vi "ADC Read Current.vi"(4 "Range":string, 8 "Bit depth":u8 max=3 step=1, 11 "VISA Refnum in":refnum<visa-resource-name>) -> (0 "Current in uA":dbl, 1 "Configuration byte":u8, 3 "VISA Refnum out":refnum<visa-resource-name>)   [LabVIEW 2015]
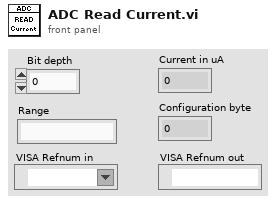
[diagram p1: front panel]
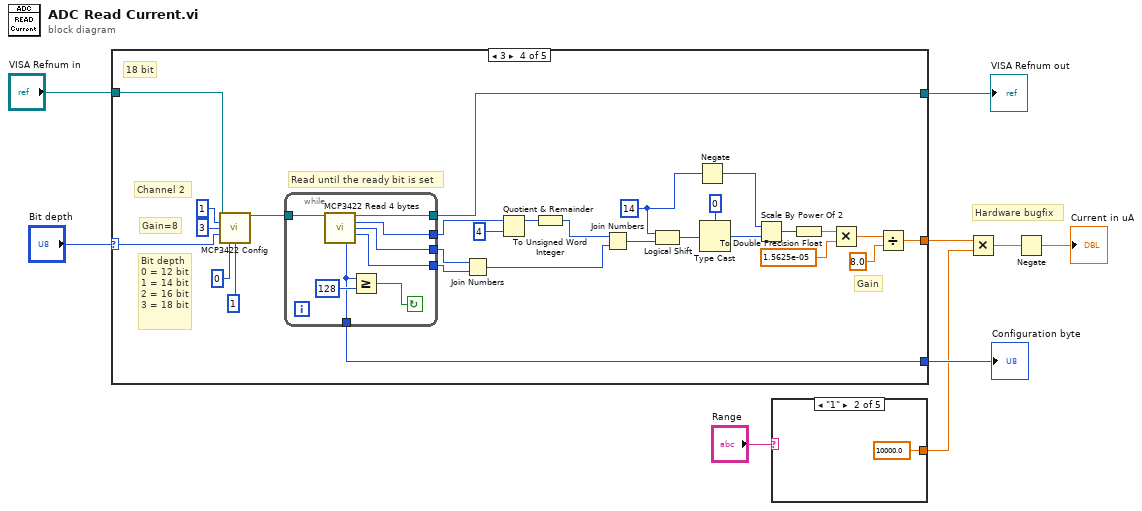
[diagram p0: block diagram]
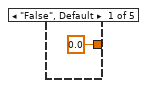
[diagram p2: hidden frame]
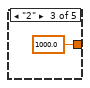
[diagram p3: hidden frame]
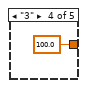
[diagram p4: hidden frame]
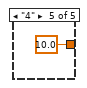
[diagram p5: hidden frame]
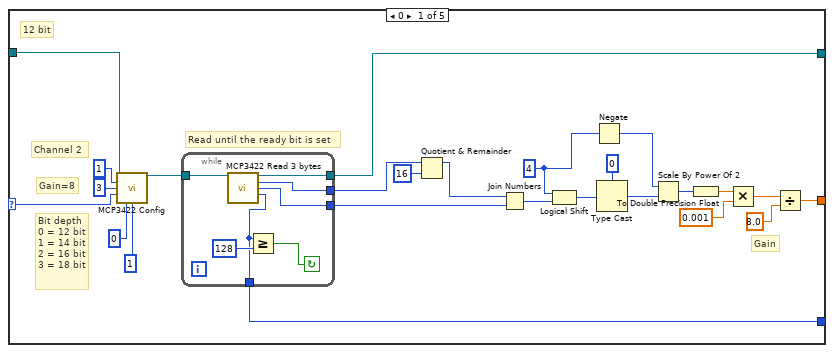
[diagram p6: hidden frame]
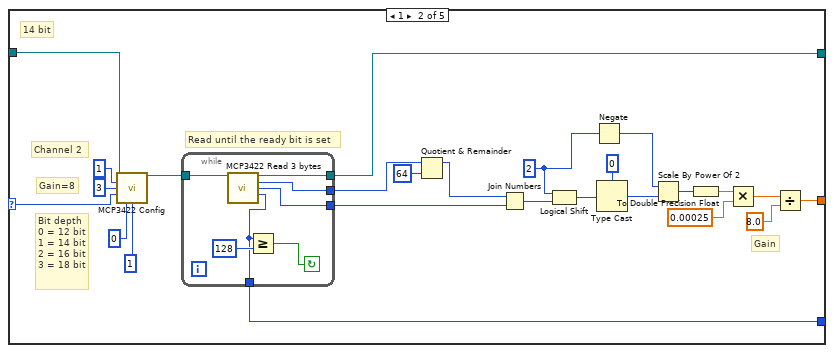
[diagram p7: hidden frame]
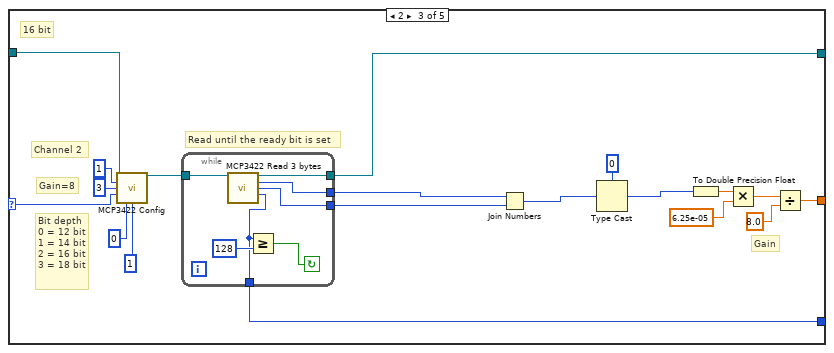
[diagram p8: hidden frame]
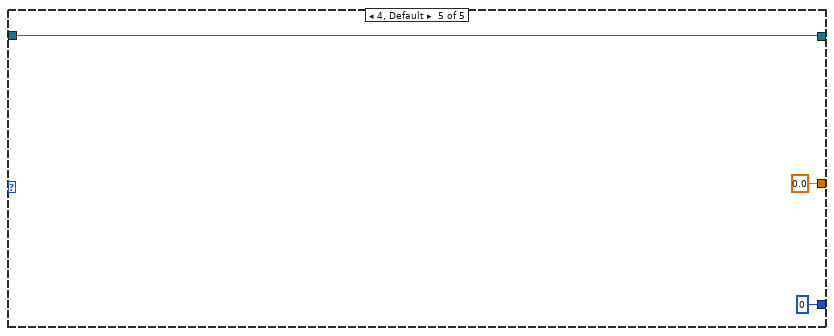
[diagram p9: hidden frame]
diagram:
  # "Hardware bugfix"
  n1 = case shown="3" "Bit depth" {
    selector: "Bit depth" -> [w17 w49 w81 w102 _]
    tunnel: "VISA Refnum in" -> [w18 w50 w82 w104 w138]
    tunnel: [w15 w47 w79 w103 w138] -> w8
    tunnel: [w16 w48 w80 w101 0.0] -> w5
    tunnel: [w10 w42 w74 w100 u8 0 ("configuration byte")] -> w6
    frame 0 {
      w22 = i16 4 ("y")
      # "Bit depth\n0 = 12 bit\n1 = 14 bit\n2 = 16 bit\n3 = 18 bit"
      # "12 bit"
      # "Gain"
      # "Read until the ready bit is set"
      # "Gain=8"
      # "Channel 2"
      n2 = call "MCP3422 Config.vi"("VISA Refnum in"=w18, "Channel selection"=u8 1, "Gain selection"=u8 3, "Sample rate selection"=w17, "Continuous conversion"=u8 0, "Initiate conversion"=u8 1) -> ("VISA Refnum out"=w30:refnum<visa-resource-name>)  [unwired: 8 in, 1 out]
      n3 = while {
        tunnel: w30 -> [w39]
        tunnel: [w38] -> w15
        tunnel: [w37] -> w12
        tunnel: [w36] -> w14
        tunnel: [w35] -> w10
        stop <- w40 continue-if-true
        n4 = call "MCP3422 Read 3 bytes.vi"("VISA Refnum in"=w39) -> ("VISA Refnum out"=w38:refnum<visa-resource-name>, "1st data byte"=w37:u8, "2nd data byte"=w36:u8, "configuration byte"=w35:u8)  [unwired: 10 in, 1 out]
        n5 = Greater Or Equal?(x=w35, y=u8 128) -> (x >= y?=w40:bool)
      }
      n6 = Quotient & Remainder(x=w12, y=u8 16) -> (x-y*floor(x/y)=w13:u8)  [unwired: 1 out]
      n7 = Join Numbers(hi=w13, lo=w14) -> ((hi.lo)=w26:u16)
      n8 = Logical Shift(y=w22, x=w26) -> (x << y=w24:u16)
      n9 = Negate(x=w22) -> (-x=w19:i16)
      n10 = Type Cast(type=i16 0, x=w24) -> (*(type *) &x=w23:i16)
      n11 = Scale By Power Of 2(n=w19, x=w23) -> (x*2^n=w21:i16)
      n12 = To Double Precision Float(number=w21) -> (double precision float=w20:dbl)
      n13 = Multiply(x=w20, y=0.001) -> (x*y=w28:dbl)
      n14 = Divide(x=w28, y=8.0) -> (x/y=w16:dbl)
    }
    frame 1 {
      w54 = i16 2 ("y")
      # "Bit depth\n0 = 12 bit\n1 = 14 bit\n2 = 16 bit\n3 = 18 bit"
      # "14 bit"
      # "Gain"
      # "Read until the ready bit is set"
      # "Gain=8"
      # "Channel 2"
      n15 = call "MCP3422 Config.vi"("VISA Refnum in"=w50, "Channel selection"=u8 1, "Gain selection"=u8 3, "Sample rate selection"=w49, "Continuous conversion"=u8 0, "Initiate conversion"=u8 1) -> ("VISA Refnum out"=w62:refnum<visa-resource-name>)  [unwired: 8 in, 1 out]
      n16 = while {
        tunnel: w62 -> [w71]
        tunnel: [w70] -> w47
        tunnel: [w69] -> w44
        tunnel: [w68] -> w46
        tunnel: [w67] -> w42
        stop <- w72 continue-if-true
        n17 = call "MCP3422 Read 3 bytes.vi"("VISA Refnum in"=w71) -> ("VISA Refnum out"=w70:refnum<visa-resource-name>, "1st data byte"=w69:u8, "2nd data byte"=w68:u8, "configuration byte"=w67:u8)  [unwired: 10 in, 1 out]
        n18 = Greater Or Equal?(x=w67, y=u8 128) -> (x >= y?=w72:bool)
      }
      n19 = Quotient & Remainder(x=w44, y=u8 64) -> (x-y*floor(x/y)=w45:u8)  [unwired: 1 out]
      n20 = Join Numbers(hi=w45, lo=w46) -> ((hi.lo)=w58:u16)
      n21 = Logical Shift(y=w54, x=w58) -> (x << y=w56:u16)
      n22 = Negate(x=w54) -> (-x=w51:i16)
      n23 = Type Cast(type=i16 0, x=w56) -> (*(type *) &x=w55:i16)
      n24 = Scale By Power Of 2(n=w51, x=w55) -> (x*2^n=w53:i16)
      n25 = To Double Precision Float(number=w53) -> (double precision float=w52:dbl)
      n26 = Multiply(x=w52, y=0.00025) -> (x*y=w60:dbl)
      n27 = Divide(x=w60, y=8.0) -> (x/y=w48:dbl)
    }
    frame 2 {
      # "Bit depth\n0 = 12 bit\n1 = 14 bit\n2 = 16 bit\n3 = 18 bit"
      # "16 bit"
      # "Gain"
      # "Read until the ready bit is set"
      # "Gain=8"
      # "Channel 2"
      n28 = call "MCP3422 Config.vi"("VISA Refnum in"=w82, "Channel selection"=u8 1, "Gain selection"=u8 3, "Sample rate selection"=w81, "Continuous conversion"=u8 0, "Initiate conversion"=u8 1) -> ("VISA Refnum out"=w88:refnum<visa-resource-name>)  [unwired: 8 in, 1 out]
      n29 = while {
        tunnel: w88 -> [w97]
        tunnel: [w96] -> w79
        tunnel: [w95] -> w77
        tunnel: [w94] -> w78
        tunnel: [w93] -> w74
        stop <- w98 continue-if-true
        n30 = call "MCP3422 Read 3 bytes.vi"("VISA Refnum in"=w97) -> ("VISA Refnum out"=w96:refnum<visa-resource-name>, "1st data byte"=w95:u8, "2nd data byte"=w94:u8, "configuration byte"=w93:u8)  [unwired: 10 in, 1 out]
        n31 = Greater Or Equal?(x=w93, y=u8 128) -> (x >= y?=w98:bool)
      }
      n32 = Join Numbers(hi=w77, lo=w78) -> ((hi.lo)=w76:u16)
      n33 = Type Cast(type=i16 0, x=w76) -> (*(type *) &x=w75:i16)
      n34 = To Double Precision Float(number=w75) -> (double precision float=w83:dbl)
      n35 = Multiply(x=w83, y=6.25e-05) -> (x*y=w86:dbl)
      n36 = Divide(x=w86, y=8.0) -> (x/y=w80:dbl)
    }
    frame 3 {
      w108 = i16 14 ("y")
      # "Bit depth\n0 = 12 bit\n1 = 14 bit\n2 = 16 bit\n3 = 18 bit"
      # "18 bit"
      # "Gain"
      # "Read until the ready bit is set"
      # "Gain=8"
      # "Channel 2"
      n37 = call "MCP3422 Config.vi"("VISA Refnum in"=w104, "Channel selection"=u8 1, "Gain selection"=u8 3, "Sample rate selection"=w102, "Continuous conversion"=u8 0, "Initiate conversion"=u8 1) -> ("VISA Refnum out"=w123:refnum<visa-resource-name>)  [unwired: 8 in, 1 out]
      n38 = while {
        tunnel: w123 -> [w133]
        tunnel: [w132] -> w103
        tunnel: [w131] -> w120
        tunnel: [w130] -> w122
        tunnel: [w129] -> w121
        tunnel: [w128] -> w100
        stop <- w134 continue-if-true
        n39 = call "MCP3422 Read 4 bytes.vi"("VISA Refnum in"=w133) -> ("VISA Refnum out"=w132:refnum<visa-resource-name>, "1st data byte"=w131:u8, "2nd data byte"=w130:u8, "3rd data byte"=w129:u8, "configuration byte"=w128:u8)  [unwired: 9 in, 1 out]
        n40 = Greater Or Equal?(x=w128, y=u8 128) -> (x >= y?=w134:bool)
      }
      n41 = Join Numbers(hi=w122, lo=w121) -> ((hi.lo)=w117:u16)
      n42 = Quotient & Remainder(x=w120, y=u8 4) -> (x-y*floor(x/y)=w118:u8)  [unwired: 1 out]
      n43 = To Unsigned Word Integer(number=w118) -> (unsigned 16bit integer=w116:u16)
      n44 = Join Numbers(hi=w116, lo=w117) -> ((hi.lo)=w112:u32)
      n45 = Logical Shift(y=w108, x=w112) -> (x << y=w110:u32)
      n46 = Negate(x=w108) -> (-x=w105:i16)
      n47 = Type Cast(type=0, x=w110) -> (*(type *) &x=w109:i32)
      n48 = Scale By Power Of 2(n=w105, x=w109) -> (x*2^n=w107:i32)
      n49 = To Double Precision Float(number=w107) -> (double precision float=w106:dbl)
      n50 = Multiply(x=w106, y=1.5625e-05) -> (x*y=w114:dbl)
      n51 = Divide(x=w114, y=8.0) -> (x/y=w101:dbl)
    }
    frame 4, Default {
    }
  }
  "VISA Refnum out" <- w8
  "Configuration byte" <- w6
  n52 = case shown="\"1\"" "Range" {
    tunnel: [0.0 10000.0 1000.0 100.0 10.0] -> w3
    frame "False", Default {
    }
    frame "1" {
    }
    frame "2" {
    }
    frame "3" {
    }
    frame "4" {
    }
  }
  n53 = Multiply(x=w5, y=w3) -> (x*y=w2:dbl)
  n54 = Negate(x=w2) -> (-x=→"Current in uA":dbl)
